vi "DAQ_Histeresis.vi"() -> ()   [LabVIEW 2020]
panel:
  in  "ValorMenor":dbl=25.0
  in  "ValorMayor":dbl=27.0
  out "element":dbl
  out "Boolean":bool
  in  "stop":bool
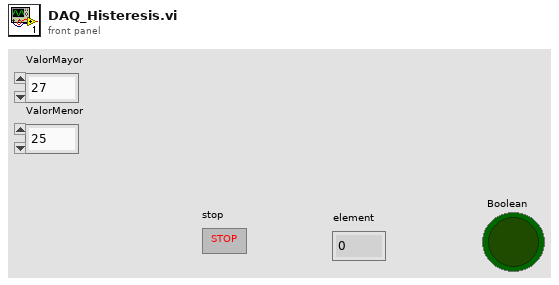
[diagram p1: front panel]
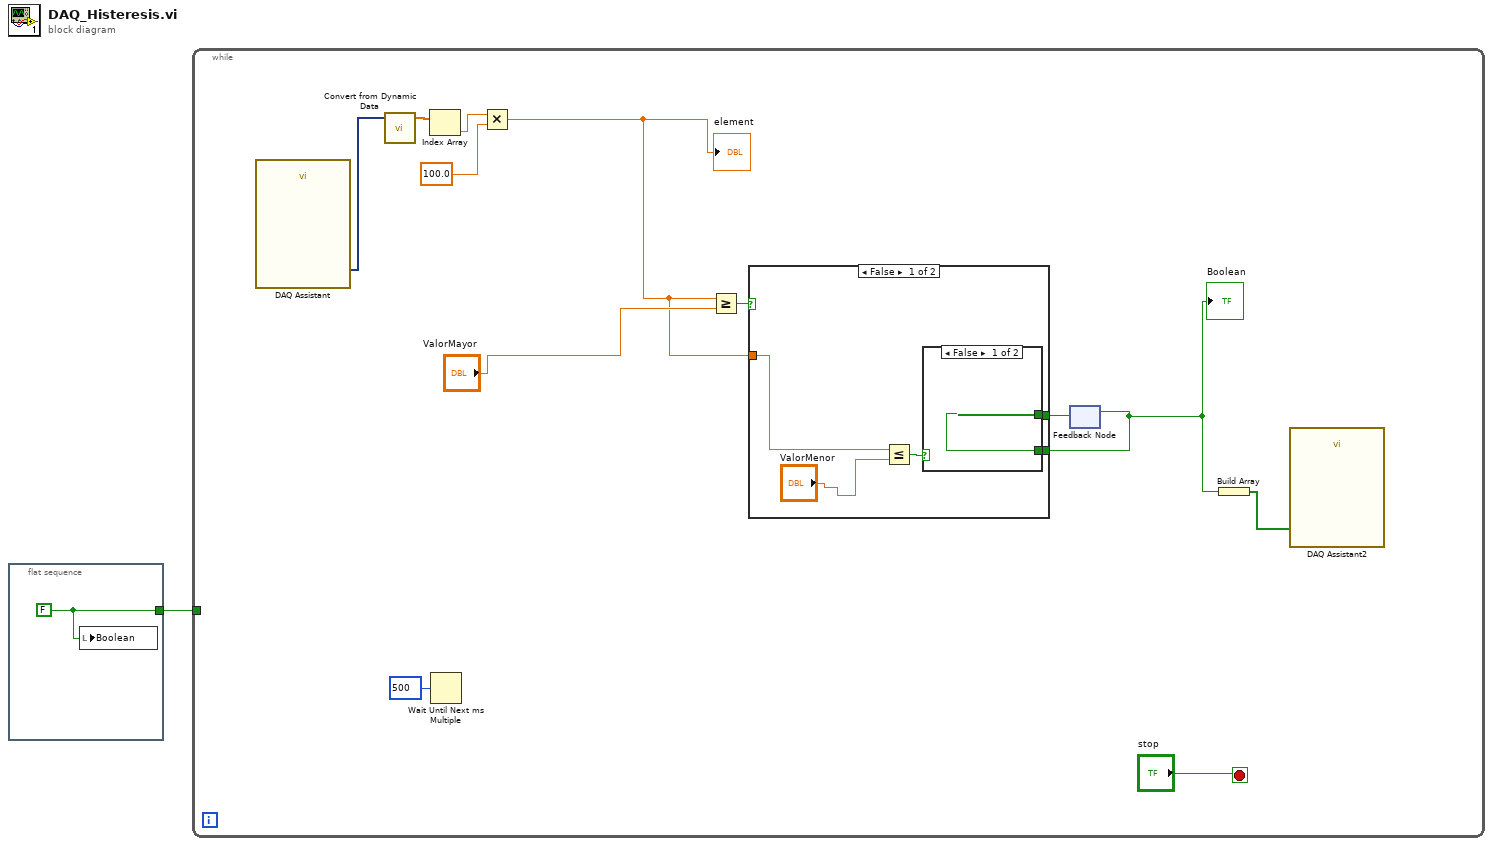
[diagram p0: block diagram]
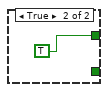
[diagram p2: hidden frame]
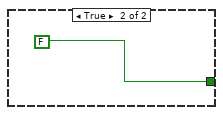
[diagram p3: hidden frame]
diagram:
  n1 = flat-sequence {
    tunnel: [w2] -> w1
    frame #0 {
      w2 = FALSE
      n2 = local write "Boolean"(w2) -> ()
    }
  }
  n3 = while {
    tunnel: w1 -> [_]
    stop <- "stop" stop-if-true
    n4 = call "DAQ Assistant"() -> ("data"=w14:dynamicdata)  [unwired: 17 in, 2 out]
    n5 = call "Convert from Dynamic Data"("Dynamic Data Type"=w14) -> ("Array"=w13:dbl[])  [unwired: 3 in]
    n6 = Index Array "Index Array"(array=w13) -> (element=w11:dbl)  [unwired: 1 in]
    n7 = Wait Until Next ms Multiple(millisecond multiple=u32 500) -> ()  [unwired: 1 out]
    n8 = Multiply(x=w11, y=100.0 ("element")) -> (x*y=w3:dbl)
    "element" <- w3
    n9 = Greater Or Equal?(x=w3, y="ValorMayor") -> (x >= y?=w6:bool)
    n10 = feedback #1() -> (w5:bool)  [unwired: 1 in]
    "Boolean" <- w5
    n11 = case shown="False" w6 {
      tunnel: w3 -> [w19 _]
      tunnel: [w17 FALSE] -> w7
      tunnel: w5 -> [w16 _]
      frame False {
        n12 = Less Or Equal?(x=w19, y="ValorMenor") -> (x <= y?=w18:bool)
        n13 = case shown="False" w18 {
          tunnel: [w20 TRUE] -> w17
          tunnel: w16 -> [w20 _]
          frame False {
          }
          frame True {
          }
        }
      }
      frame True {
      }
    }
    n14 = feedback-in #1(w7) -> ()
    n15 = Build Array "Build Array"(w5) -> (w9:bool[])
    n16 = call "DAQ Assistant2"("data"=w9) -> ()  [unwired: 17 in, 2 out]
  }
